vi "Add Dependent File Property Node.vi"(7 "Node Type":string, 9 "Dependent File Inputs":T1, 10 "Property Parent":string, 11 "Doc Ref":refnum<k20>) -> (1 "Updated Node Ref":refnum<k20>, 3 "Node Found?":bool)   [LabVIEW 2025]
uses:
  <resource>/objmgr/DOMUserDefRef.rc
  Shared/Types/NodeFilteringOptions.ctl
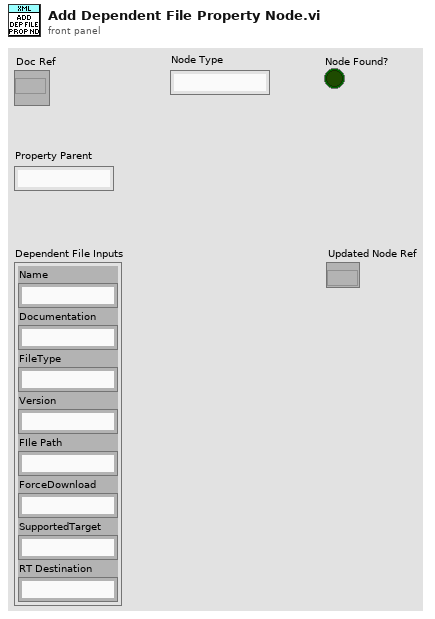
[diagram p1: front panel]
types:
  T1 = cluster{"Name":string, "Documentation":string, "FileType":string, "Version":string, "FIle Path":string, "ForceDownload":string, "SupportedTarget":string, "RT Destination":string}
  T2 = typedef "NodeFilteringOptions.ctl" = enum16{"GetCustomDeviceNode", "GetAllChannelNodes", "GetAllSectionNodes", "GetAllWaveformNodes", "GetFirstChannelNode", "GetFirstSectionNode", "GetFirstWaveformNode", "GetSpecificSectionNode", "GetSpecificCustomDeviceNode", "GetSpecificChannelNode", "GetSpecificWaveformNode", "GetMatchedNamedNode", "GetEnumDefinitionsNode", "GetSpecificEnumDefinitionNode", "GetAllEnumDefinitionNodes", "GetDynamicChannelNodes"}
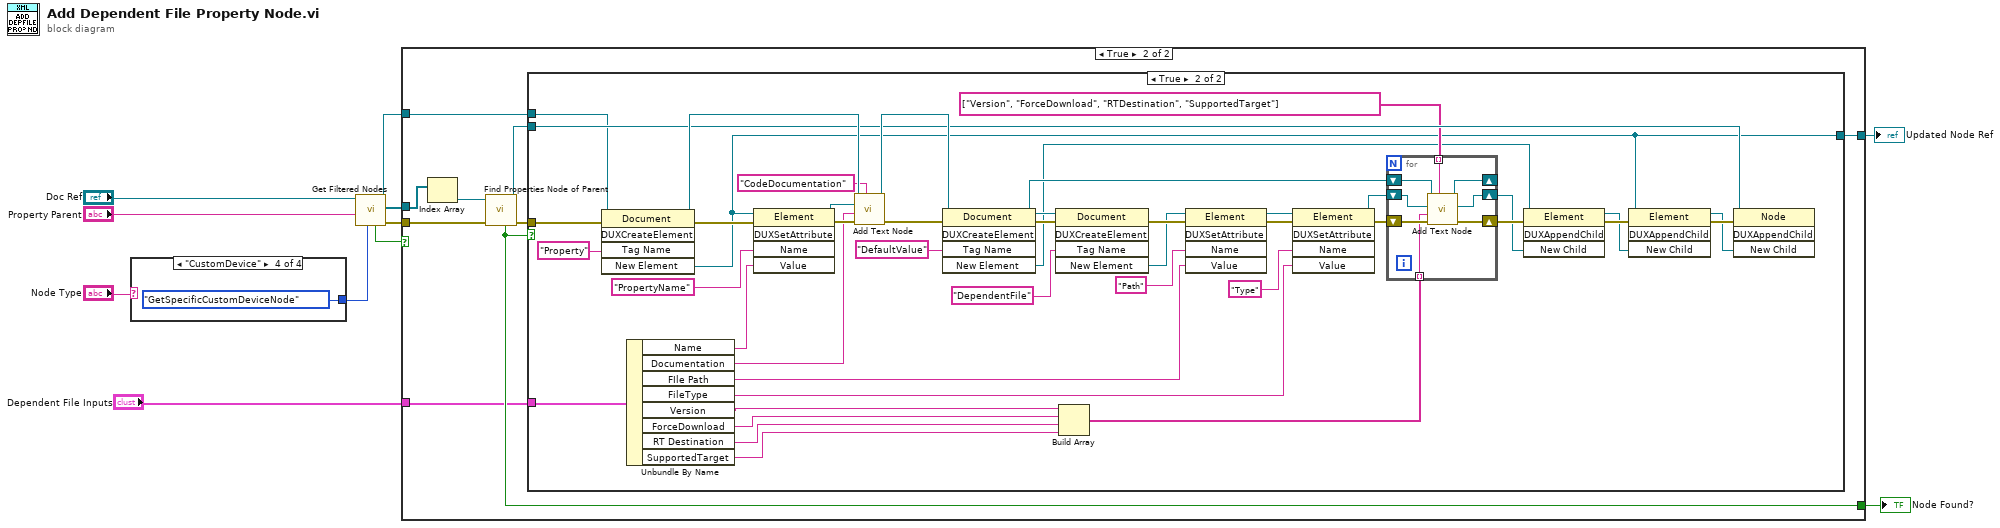
[diagram p0: block diagram]
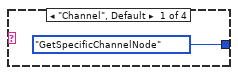
[diagram p4: hidden frame]
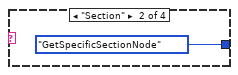
[diagram p5: hidden frame]
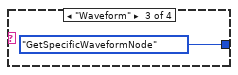
[diagram p6: hidden frame]
diagram:
  n1 = case shown="\"CustomDevice\"" "Node Type" {
    tunnel: [NodeFilteringOptions."GetSpecificChannelNode" ("Node Filtering") NodeFilteringOptions."GetSpecificSectionNode" ("Node Filtering") NodeFilteringOptions."GetSpecificWaveformNode" ("Node Filtering") NodeFilteringOptions."GetSpecificCustomDeviceNode" ("Node Filtering")] -> w9
    frame "Channel", Default {
    }
    frame "Section" {
    }
    frame "Waveform" {
    }
    frame "CustomDevice" {
    }
  }
  n2 = call "Get Filtered Nodes.vi"("Node Filtering"=w9, "Node Name"="Property Parent", "Document in"="Doc Ref") -> ("error out"=w7:errorcluster, "Filtered Nodes"=w4:refnum<k20>[], "Document out"=w6:refnum<k20>, "Node Found?"=w5:bool)  [unwired: 4 in, 1 out]
  n3 = case shown="True" w5 {
    tunnel: [_ w22] -> w11
    tunnel: w7 -> [_ w21]
    tunnel: w6 -> [_ w20]
    tunnel: w4 -> [_ w19]
    tunnel: "Dependent File Inputs" -> [_ w17]
    tunnel: [_ w16] -> w1
    frame False {
    }
    frame True {
      n4 = Index Array(array=w19) -> (element=w18:refnum<k20>)  [unwired: 1 in]
      n5 = call "Find Properties Node of Parent.vi"("error in"=w21, "Node"=w18) -> ("error out"=w23:errorcluster, "Poperties Node"=w24:refnum<k20>, "Node Found?"=w22:bool)  [unwired: 7 in]
      n6 = case shown="True" w22 {
        tunnel: w24 -> [_ w58]
        tunnel: w23 -> [_ w56]
        tunnel: w20 -> [_ w55]
        tunnel: w17 -> [_ w54]
        tunnel: [_ w25] -> w16
        frame False {
        }
        frame True {
          n7 = invoke class="Document" method="DUXCreateElement"(reference=w55, error in=w56, "Tag Name"="Property") -> (reference out=w63:refnum<k20>, error out=w67:errorcluster, "New Element"=w25:refnum<k20>)  [unwired: 2 in, 2 out]
          n8 = Unbundle By Name(w54) -> ("Name"=w53:string, "Documentation"=w52:string, "FIle Path"=w45:string, "FileType"=w41:string, "Version"=w38:string, "ForceDownload"=w37:string, "RT Destination"=w36:string, "SupportedTarget"=w35:string)
          n9 = invoke class="Element" method="DUXSetAttribute"(reference=w25, error in=w67, "Name"="PropertyName", "Value"=w53) -> (reference out=w62:refnum<k20>, error out=w66:errorcluster)  [unwired: 1 in, 3 out]
          n10 = call "Add Text Node.vi"("Tag Name"="CodeDocumentation", "error in"=w66, "Tag Data"=w52, "Element in"=w62, "Document in"=w63) -> ("error out"=w59:errorcluster, "Document out"=w61:refnum<k20>)  [unwired: 4 in, 1 out]
          n11 = invoke class="Document" method="DUXCreateElement"(reference=w61, error in=w59, "Tag Name"="DefaultValue") -> (reference out=w50:refnum<k20>, error out=w51:errorcluster, "New Element"=w27:refnum<k20>)  [unwired: 2 in, 2 out]
          n12 = invoke class="Document" method="DUXCreateElement"(reference=w50, error in=w51, "Tag Name"="DependentFile") -> (error out=w48:errorcluster, "New Element"=w47:refnum<k20>)  [unwired: 2 in, 3 out]
          n13 = Build Array(w38, w37, w36, w35) -> (w34:string[])
          n14 = invoke class="Element" method="DUXSetAttribute"(reference=w47, error in=w48, "Name"="Path" ("Tag Name"), "Value"=w45) -> (reference out=w43:refnum<k20>, error out=w44:errorcluster)  [unwired: 1 in, 3 out]
          n15 = invoke class="Element" method="DUXSetAttribute"(reference=w43, error in=w44, "Name"="Type" ("Tag Name"), "Value"=w41) -> (reference out=w33:refnum<k20>, error out=w40:errorcluster)  [unwired: 1 in, 3 out]
          n16 = for {
            shift-right: [w73] -> _
            shift-left: w50 -> [w75]
            shift-right: [w71] -> w31
            shift-left: w33 -> [w72]
            tunnel: string[] ["Version", "ForceDownload", "RTDestination", "SupportedTarget"] -> [w70] mode=indexing
            tunnel: w34 -> [w69] mode=indexing
            shift-right: [w68] -> w32
            shift-left: w40 -> [w74]
            n17 = call "Add Text Node.vi"("Tag Name"=w70, "error in"=w74, "Tag Data"=w69, "Element in"=w72, "Document in"=w75) -> ("error out"=w68:errorcluster, "Element out"=w71:refnum<k20>, "Document out"=w73:refnum<k20>)  [unwired: 4 in]
          }
          n18 = invoke class="Element" method="DUXAppendChild"(reference=w27, error in=w32, "New Child"=w31) -> (reference out=w26:refnum<k20>, error out=w30:errorcluster)  [unwired: 1 in, 2 out]
          n19 = invoke class="Element" method="DUXAppendChild"(reference=w25, error in=w30, "New Child"=w26) -> (reference out=w28:refnum<k20>, error out=w29:errorcluster)  [unwired: 1 in, 2 out]
          n20 = invoke class="Node" method="DUXAppendChild"(reference=w58, error in=w29, "New Child"=w28) -> ()  [unwired: 1 in, 4 out]
        }
      }
    }
  }
  "Node Found?" <- w11
  "Updated Node Ref" <- w1
